vi "process.vi"(8 "error in (no error)":errorcluster, 9 "Calling VI Reference i":refnum<vi>, 10 "Node Refnum":refnum<vi>, 11 "DefaultNode in":refnum<class "DefaultNode.lvclass">) -> (0 "error out":errorcluster, 3 "DefaultNode out":refnum<class "DefaultNode.lvclass">)   [LabVIEW 2016, in "DefaultNode.lvclass"]
uses:
  DefaultNode.lvclass
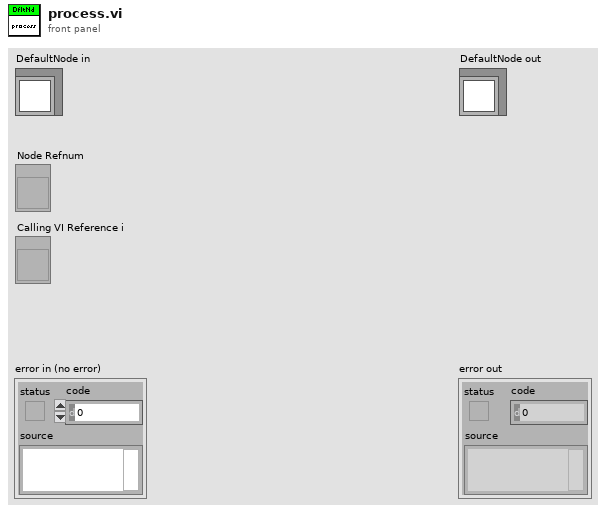
[diagram p1: front panel]
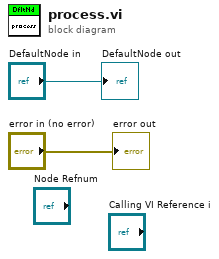
[diagram p0: block diagram]
diagram:
  "error out" <- "error in (no error)"
  "DefaultNode out" <- "DefaultNode in"
